vi "Lang Get PC Language.vi"() -> (3 "Language Hex Code":string)   [LabVIEW 2018, in "Framework.lvlib" / "Framework.lvclass"]
uses:
  Framework.lvclass
  kernel32.dll
panel:
  out "LanguageID":i32 format="%.0x"
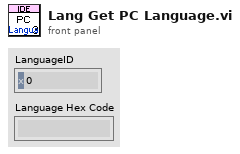
[diagram p1: front panel]
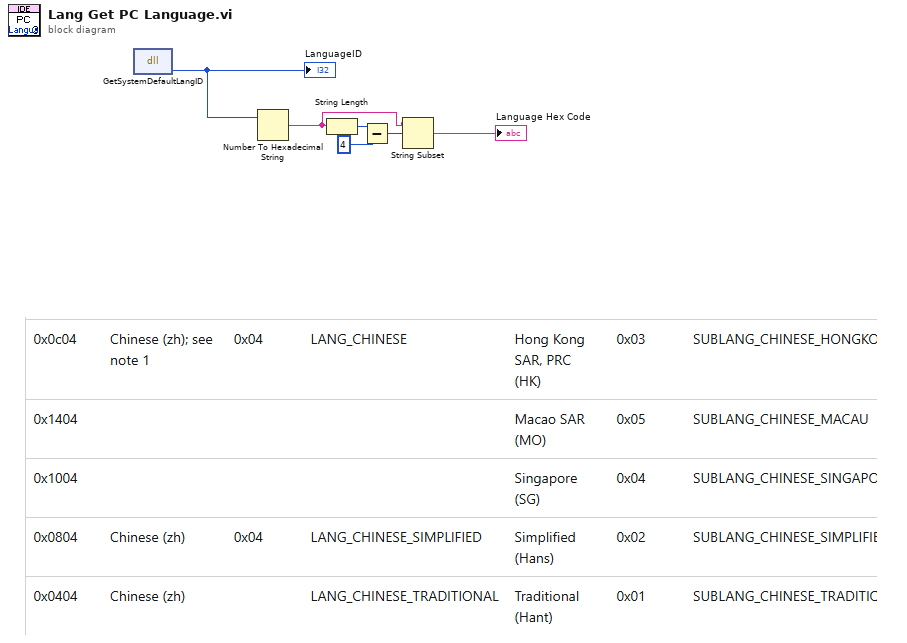
[diagram p0: block diagram]
diagram:
  n1 = dll-call lib="kernel32.dll" fn="GetSystemDefaultLangID"() -> ("LanguageID"=w6:i32)  [unwired: 3 in, 2 out]
  "LanguageID" <- w6
  n2 = Number To Hexadecimal String(2:w6) -> (0:w2:string)  [unwired: 1 in]
  n3 = String Length(string=w2) -> (length=w5:i32)
  n4 = Subtract(x=w5, y=4) -> (x-y=w3:i32)
  n5 = String Subset(string=w2, offset (0)=w3) -> (substring=→"Language Hex Code":string)  [unwired: 1 in]
